vi "PCI1716.vi"(9 "退出？":bool) -> ()   [LabVIEW 2010]
panel:
  out "灯":bool[](array[boolean])
  out "布尔":bool
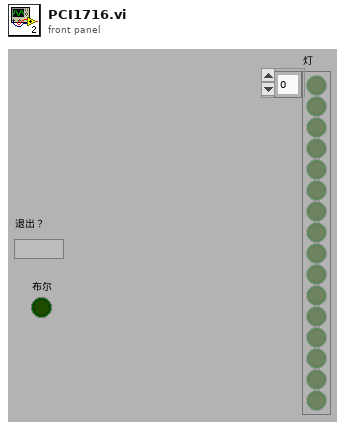
[diagram p1: front panel]
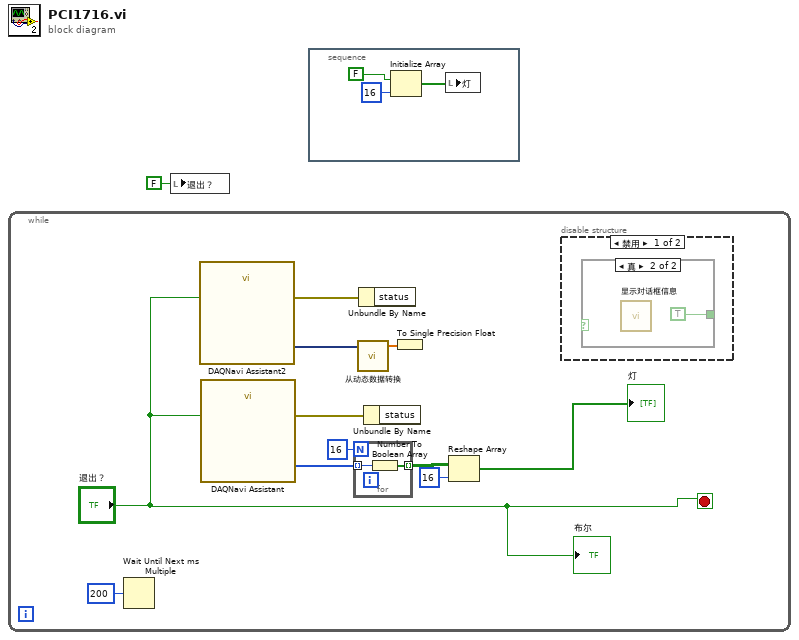
[diagram p0: block diagram]
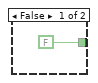
[diagram p2: hidden frame]
diagram:
  n1 = while {
    stop <- "退出？" stop-if-true
    n2 = Wait Until Next ms Multiple(millisecond multiple=u32 200 ("毫秒倍数")) -> ()  [unwired: 1 out]
    n3 = call "DAQNavi Assistant2"("stop(true)"="退出？") -> ("error out"=w5:errorcluster, "data out(DDT)"=w4:dynamicdata)  [unwired: 1 in, 16 out]
    n4 = call "DAQNavi Assistant"("stop(true)"="退出？") -> ("error out"=w8:errorcluster, "dataOut(U8Array)"=w12:u8[])  [unwired: 1 in, 16 out]
    n5 = for {
      N: 16 -> [_]
      tunnel: [w16] -> w11 mode=indexing
      tunnel: w12 -> [w15] mode=indexing
      n6 = Number To Boolean Array(number=w15) -> (Boolean array=w16:bool[])
    }
    n7 = call "从动态数据转换"("Dynamic Data Type"=w4) -> ("Array"=w3:dbl[])  [unwired: 3 in]
    n8 = Unbundle By Name(w5) -> ()  [unwired: 1 out]
    n9 = Unbundle By Name(w8) -> ()  [unwired: 1 out]
    n10 = To Single Precision Float(number=w3) -> ()  [unwired: 1 out]
    n11 = Reshape Array(w11, 16 ("维数大小")) -> (→"灯":bool[])
    n12 = disable-structure shown="禁用" {
      frame Disabled {
        n13 = case shown="真" {
          selector: _ -> [_ _]
          tunnel: [FALSE TRUE] -> _
          frame False {
          }
          frame True {
            n14 = call "显示对话框信息"() -> ()  [unwired: 10 in, 2 out]
          }
        }
      }
      frame Enabled {
      }
    }
    "布尔" <- "退出？"
  }
  n15 = local write "退出？"(FALSE ("退出？")) -> ()
  n16 = stacked-sequence {
    frame #0 {
      n17 = Initialize Array(FALSE, 16 ("维数大小")) -> (w17:bool[])
      n18 = local write "灯"(w17) -> ()
    }
  }
